vi "Write temperature.vi"(8 "error in (no error)":errorcluster, 10 "temperature":dbl=1.0, 11 "abstract_llm_base in":refnum<class "abstract_llm_base.lvclass">) -> (0 "error out":errorcluster, 3 "abstract_llm_base out":refnum<class "abstract_llm_base.lvclass">)   [LabVIEW 2020, in "abstract_llm_base.lvclass"]
uses:
  abstract_llm_base.lvclass
  abstract_llm_base.lvclass/abstract_llm_base.ctl
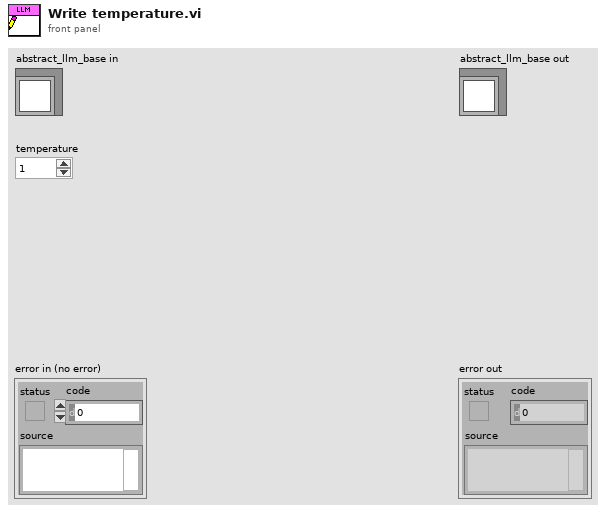
[diagram p1: front panel]
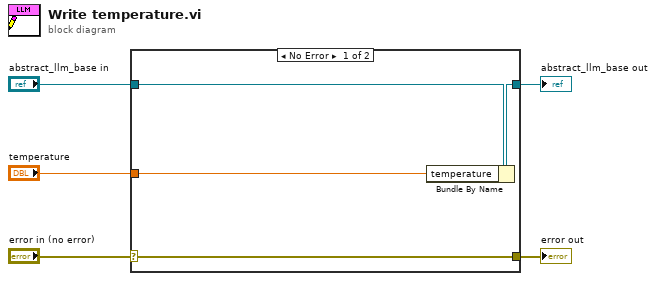
[diagram p0: block diagram]
diagram:
  n1 = case shown="No Error" "error in (no error)" {
    selector: "error in (no error)" -> [w9 w10]
    tunnel: [w9 w10] -> w4
    tunnel: [w7 w11] -> w2
    tunnel: "abstract_llm_base in" -> [w8 w11]
    tunnel: "temperature" -> [w6 _]
    frame No Error {
      n2 = Bundle By Name(cluster=w8, "temperature"=w6) -> (w7:refnum<class "abstract_llm_base.lvclass">)
    }
    frame Error {
    }
  }
  "error out" <- w4
  "abstract_llm_base out" <- w2
